vi "Histogram Avoidance.vi"(8 "Error In":errorcluster, 11 "Control":T2={"Max speed (m/s)"=0.4, "Inner threshold"=0.6, "Outer threshold"=1.1, "Data (deg) (m)"=[], "Initialize?"=FALSE, "Distance (m)"=0.0, "Obstacle clearance (m)"=1.0, "Current heading (deg)"=0.0} {"Current heading (deg)" scale=-180.0..180.0}) -> (0 "Error Out":errorcluster, 3 "Output":T1)   [LabVIEW 2011]
uses:
  <vilib>/robotics/Controls/Compass Indicator/Compass Indicator.xctl
  <vilib>/Analysis/coordinate.llb/Angle Range (Degree).ctl
  <vilib>/Analysis/coordinate.llb/Angle Units.ctl
  <vilib>/Analysis/coordinate.llb/Wrap Angle (scalar).vi
  <vilib>/Analysis/NI_AAL_Angle.lvlib
panel:
  out "mask out":bool[](array[boolean])
  out "Obstacle clearance (m)":dbl=1.0
  out "Command heading":dbl(xcontrol)
  out "Current heading":dbl(xcontrol)
  in  "Initialize?":bool
  out "heading 180":dbl(slide) scale=-180.0..180.0
  out "Desired heading (deg)":dbl(slide) scale=-180.0..180.0
  out "Mask":i16[](graph)
  out "Distance (m)":dbl
  out "Data (deg) (m)":dbl[][](array[numeric])
  out "command vx":dbl
  out "command vy":dbl
  out "command heading (deg)":dbl
  out "command heading (rad)":dbl
  out "histogram out":dbl[](graph)
  out "Outer threshold":dbl=1.1
  out "Inner threshold":dbl=0.6
  out "Max speed (m/s)":dbl=0.4
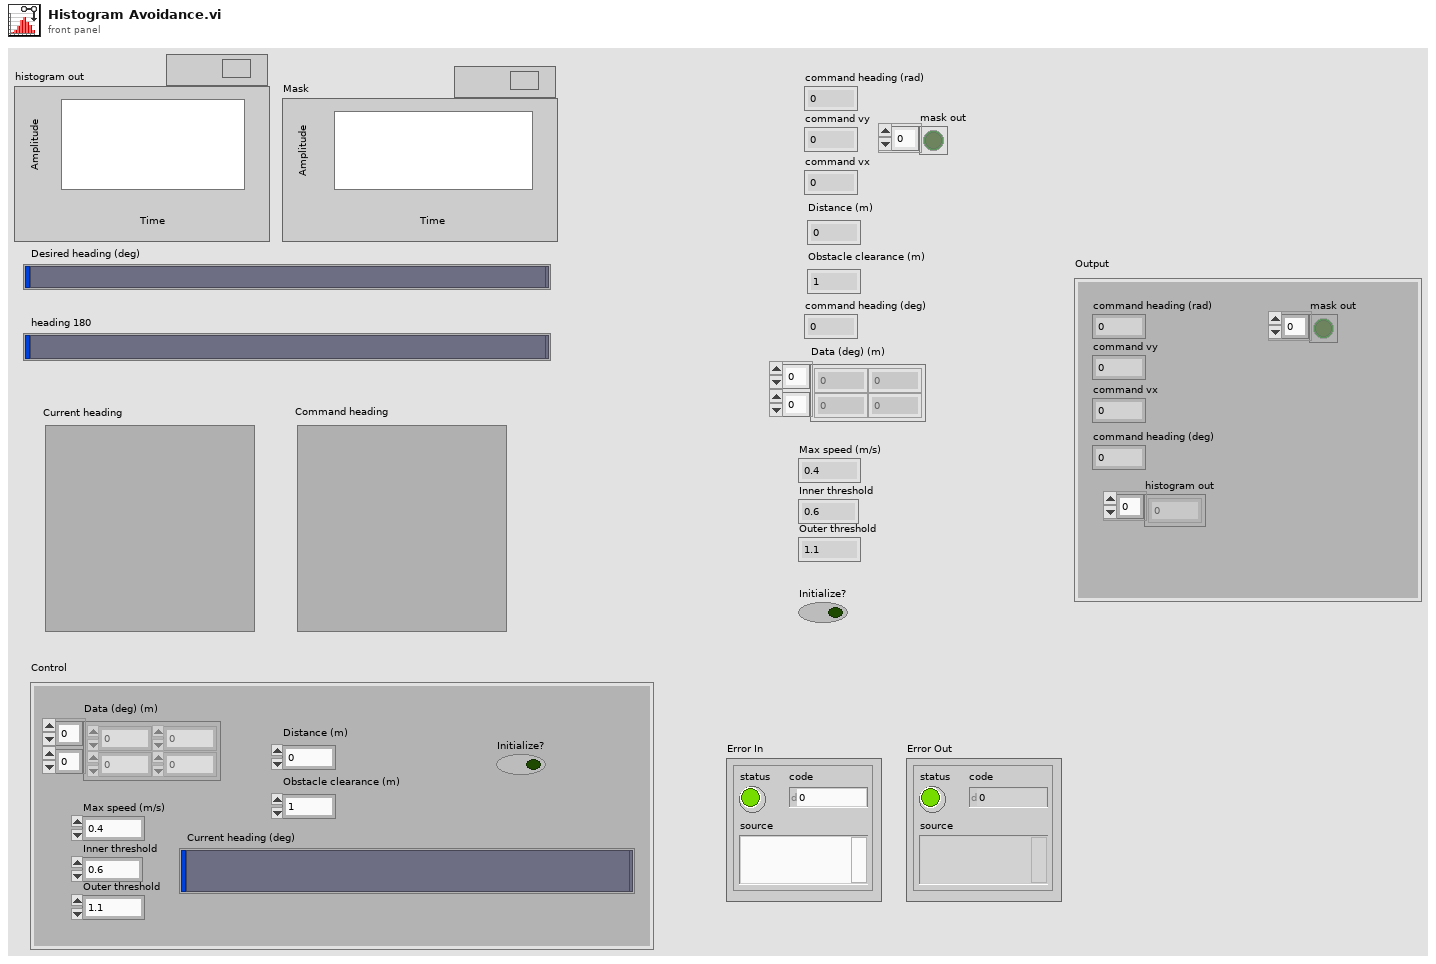
[diagram p1: front panel]
types:
  T1 = cluster{"command heading (rad)":dbl, "command vy":dbl, "command vx":dbl, "mask out":bool[], "command heading (deg)":dbl, "histogram out":dbl[]}
  T2 = cluster{"Max speed (m/s)":dbl, "Inner threshold":dbl, "Outer threshold":dbl, "Data (deg) (m)":dbl[][], "Initialize?":bool, "Distance (m)":dbl, "Obstacle clearance (m)":dbl, "Current heading (deg)":dbl}
  T3 = typedef "NI_AAL_Angle.lvlib/Angle Units.ctl" = i32
  T4 = typedef "NI_AAL_Angle.lvlib/Angle Range (Degree).ctl" = u16
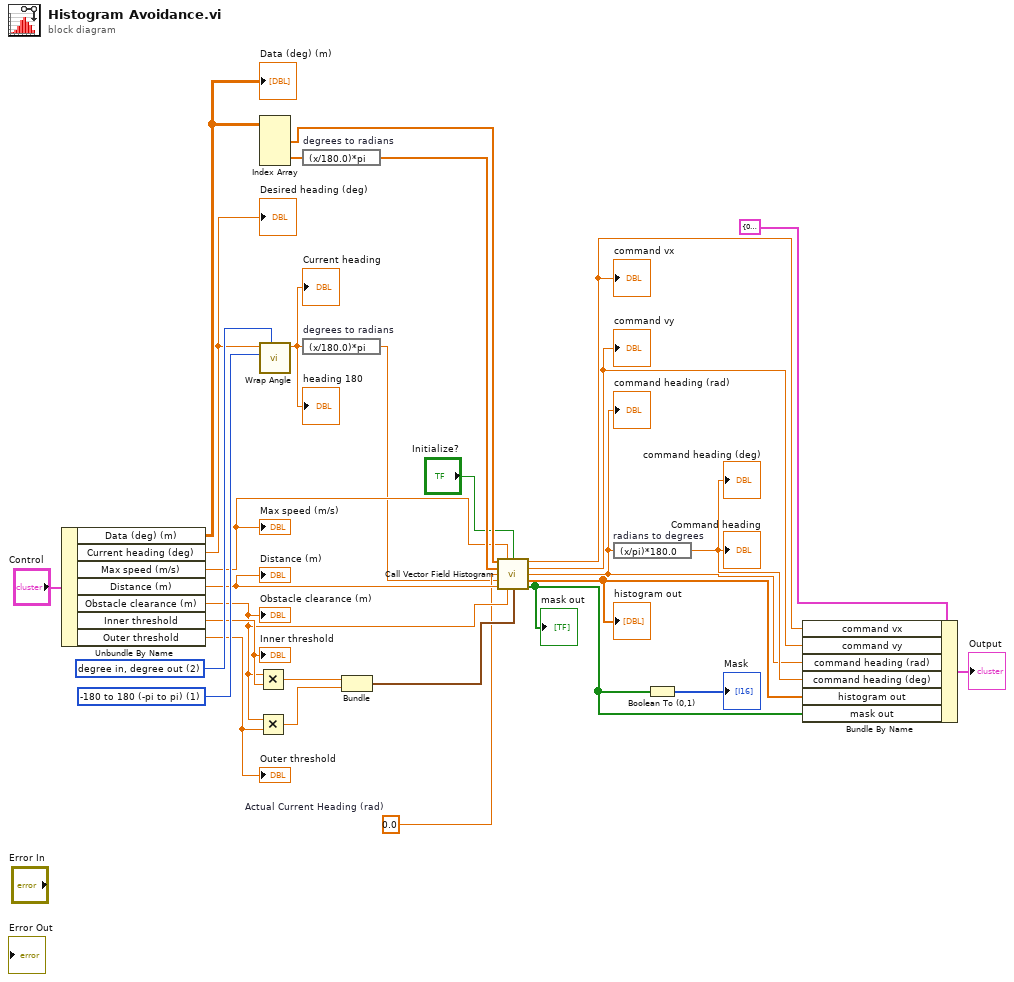
[diagram p0: block diagram]
diagram:
  w21 = T3 2 items=["radian in, radian out", "radian in, degree out", "degree in, degree out", "degree in, radian out"] ("angle units")
  w22 = T4 1 items=["none", "-180 to 180 (-pi to pi)", "0 to 360 (0 to 2pi)"] ("angle range")
  w2 = 0.0  # Actual Current Heading (rad)
  n1 = Unbundle By Name("Control") -> ("Data (deg) (m)"=w11:dbl[][], "Current heading (deg)"=w12:dbl, "Max speed (m/s)"=w13:dbl, "Distance (m)"=w14:dbl, "Obstacle clearance (m)"=w15:dbl, "Inner threshold"=w16:dbl, "Outer threshold"=w17:dbl)
  "Max speed (m/s)" <- w13
  "Inner threshold" <- w16
  "Outer threshold" <- w17
  "Data (deg) (m)" <- w11
  "Distance (m)" <- w14
  "Desired heading (deg)" <- w12
  "Obstacle clearance (m)" <- w15
  n2 = Multiply(x=w15, y=w16) -> (x*y=w29:dbl)
  n3 = Multiply(x=w15, y=w17) -> (x*y=w28:dbl)
  n4 = Index Array(array=w11) -> (element #1=w26:dbl[], element #2=w24:dbl[])  [unwired: 4 in]
  n5 = call-poly <vilib>:"Wrap Angle.vi"("angle units"=w21, "angle range"=w22, "angle in"=w12) -> ("angle out"=w19:dbl)  [unwired: 7 in, 1 out]
  "heading 180" <- w19
  "Current heading" <- w19
  n6 = expression code="(x/180.0)*pi" "degrees to radians"(w24) -> (w23:dbl[])
  n7 = expression code="(x/180.0)*pi" "degrees to radians"(w19) -> (w1:dbl)
  n8 = Bundle(w29, w28) -> (w27:cluster{dbl, dbl})  [unwired: 1 in]
  n9 = call "Call Vector Field Histogram.vi"("LIDAR magn. (m)"=w26, "max speed"=w13, "Initialize?"="Initialize?", "LIDAR angle (rad)"=w23, "current heading (rad)"=w2, "target heading (rad)"=w1, "target distance"=w14, "obstacle clearance (m)"=w15, "thresholds"=w27) -> ("command vx"=w10:dbl, "command vy"=w9:dbl, "command heading (rad)"=w3:dbl, "histogram out"=w5:dbl[], "mask out"=w4:bool[])  [unwired: 2 in]
  "histogram out" <- w5
  "command heading (rad)" <- w3
  "command vy" <- w9
  "command vx" <- w10
  "mask out" <- w4
  n10 = expression code="(x/pi)*180.0" "radians to degrees"(w3) -> (w8:dbl)
  "command heading (deg)" <- w8
  "Command heading" <- w8
  n11 = Boolean To (0,1)(Boolean=w4) -> (0, 1=→"Mask":i16[])
  n12 = Bundle By Name(cluster=T1 {"command heading (rad)"=0.0, "command vy"=0.0, "command vx"=0.0, "mask out"=[], "command heading (deg)"=0.0, "histogram out"=[]} ("Cluster"), "command vx"=w10, "command vy"=w9, "command heading (rad)"=w3, "command heading (deg)"=w8, "histogram out"=w5, "mask out"=w4) -> (→"Output":T1)
